vi "Server.vi"() -> ()   [LabVIEW 2013, in "OPC UA Demo.lvlib"]
doc: "Demonstrates the use of the <B>OPC UA Server</B> VIs to programmatically create an OPC UA server."
uses:
  OPC UA Demo.lvlib
  <vilib>/OPCUA/server/subVI/supported security policies.ctl
  <vilib>/OPCUA/server/Write Int32.vi
  <vilib>/OPCUA/server/Read Int32.vi
  <vilib>/OPCUA/NI OPC UA Server.lvlib
  <vilib>/OPCUA/NI OPC UA Utility.lvlib
panel:
  out "appended array":path[](array[path])
  out "certificate path":path
  in  "supported security policies (None)":T1={"None"=TRUE, "Sign with Basic128Rsa125"=TRUE, "Sign and Encrypt with Basic128Rsa125"=TRUE, "Sign with Basic256"=TRUE, "Sign and Encrypt with Basic256"=TRUE}
  out "Device.Node.Set Point":i32
  out "Device.Node":i32
  out "server endpoint URL":string
  out "error out":errorcluster
  in  "stop":bool
  # "Overview: Demonstrates the use of the OPC UA Server VIs to programmatically create an OPC UA server.\nRequirements: \n1. LabVIEW Datalogging and Supervisory Control Module or LabVIEW Real-Time Module\n2. (Real-Time Module) RT target\nInstructions:\nRun the VI."
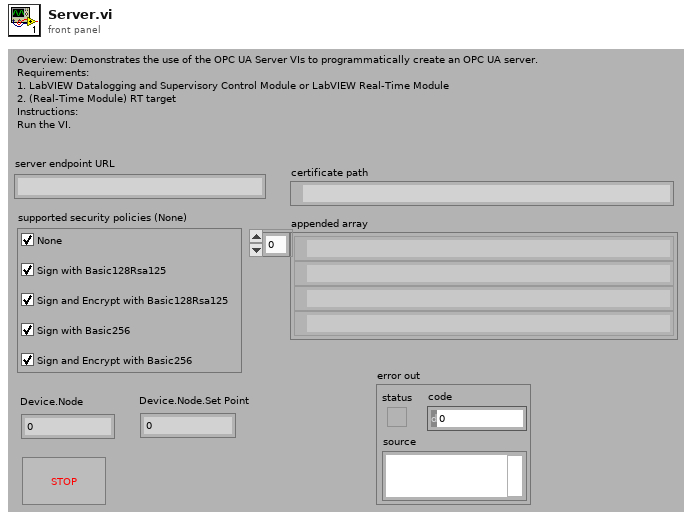
[diagram p1: front panel]
types:
  T1 = typedef "supported security policies.ctl" = cluster{"None":bool, "Sign with Basic128Rsa125":bool, "Sign and Encrypt with Basic128Rsa125":bool, "Sign with Basic256":bool, "Sign and Encrypt with Basic256":bool}
  T2 = cluster{"name":string, "data type":u16, "access level":u16, "description":string}
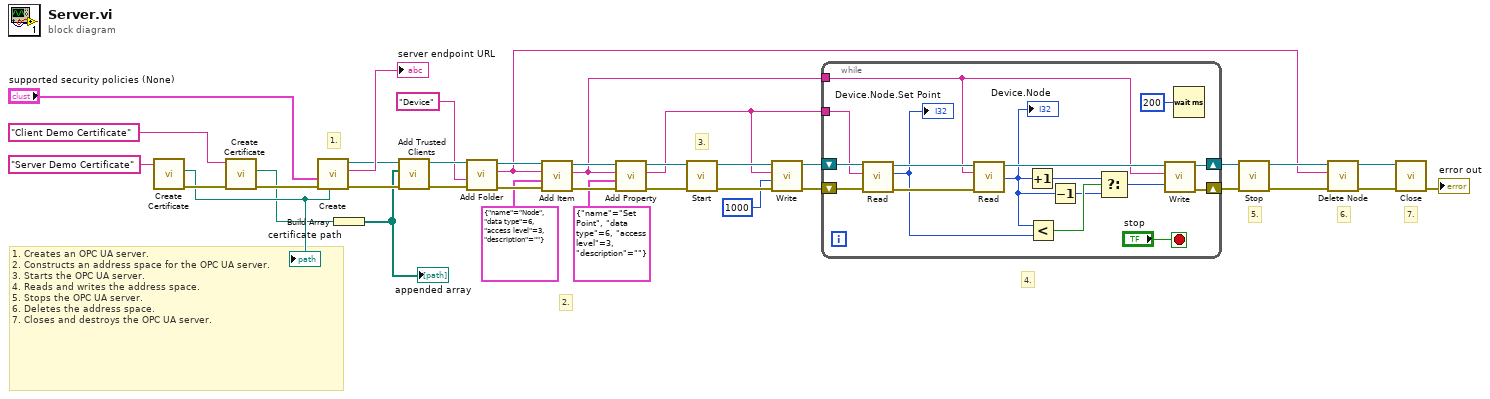
[diagram p0: block diagram]
diagram:
  # "1. Creates an OPC UA server.\n2. Constructs an address space for the OPC UA server.\n3. Starts the OPC UA server.\n4. Reads and writes the address space.\n5. Stops the OPC UA server.\n6. Deletes the address space.\n7. Closes and destroys the OPC UA server."
  # "7."
  # "6."
  # "5."
  # "4."
  # "3."
  # "2."
  # "1."
  n1 = call <vilib>:"Create Certificate.vi"("certificate name in"="Server Demo Certificate") -> ("error out"=w8:errorcluster, "certificate path"=w4:path)  [unwired: 7 in, 2 out]
  "certificate path" <- w4
  n2 = call <vilib>:"Create Certificate.vi"("error in (no error)"=w8, "certificate name in"="Client Demo Certificate") -> ("error out"=w6:errorcluster, "certificate path"=w3:path)  [unwired: 6 in, 2 out]
  n3 = call <vilib>:"Create.vi"("server certificate file"=w4, "error in (no error)"=w6, "supported security policies (None)"="supported security policies (None)") -> ("error out"=w11:errorcluster, "server endpoint URL"=→"server endpoint URL":string, "OPC UA server refnum out"=w13:refnum<k21>)  [unwired: 6 in]
  n4 = Build Array(w3) -> (w7:path[])
  "appended array" <- w7
  n5 = call <vilib>:"Add Trusted Clients.vi"("error in (no error)"=w11, "trusted client certificates"=w7, "OPC UA server refnum in"=w13) -> ("error out"=w10:errorcluster, "OPC UA server refnum out"=w12:refnum<k21>)  [unwired: 7 in]
  n6 = call <vilib>:"Add Folder.vi"("error in (no error)"=w10, "folder name"="Device", "OPC UA server refnum in"=w12) -> ("error out"=w36:errorcluster, "folder path"=w17:string, "OPC UA server refnum out"=w37:refnum<k21>)  [unwired: 5 in]
  n7 = call <vilib>:"Add Item.vi"("error in (no error)"=w36, "item"=T2 {"name"="Node", "data type"=6, "access level"=3, "description"=""}, "parent folder path"=w17, "OPC UA server refnum in"=w37) -> ("error out"=w23:errorcluster, "item path"=w1:string, "OPC UA server refnum out"=w35:refnum<k21>)  [unwired: 4 in]
  n8 = call <vilib>:"Add Property.vi"("error in (no error)"=w23, "property"=T2 {"name"="Set Point", "data type"=6, "access level"=3, "description"=""} ("item"), "item path"=w1, "OPC UA server refnum in"=w35) -> ("error out"=w22:errorcluster, "property path"=w15:string, "OPC UA server refnum out"=w24:refnum<k21>)  [unwired: 4 in]
  n9 = call <vilib>:"Start.vi"("error in (no error)"=w22, "OPC UA server refnum in"=w24) -> ("error out"=w19:errorcluster, "OPC UA server refnum out"=w34:refnum<k21>)  [unwired: 8 in]
  n10 = call-poly <vilib>:"Write.vi"("error in (no error)"=w19, "value"=1000, "node path"=w15, "OPC UA server refnum in"=w34) -> ("error out"=w18:errorcluster, "OPC UA server refnum out"=w20:refnum<k21>)  [unwired: 6 in]
  n11 = while {
    tunnel: w1 -> [w44]
    shift-right: [w50] -> w29
    shift-left: w20 -> [w49]
    shift-right: [w48] -> w27
    shift-left: w18 -> [w52]
    tunnel: w15 -> [w47]
    stop <- "stop" stop-if-true
    n12 = call-poly <vilib>:"Read.vi"("error in (no error)"=w52, "node path"=w47, "OPC UA server refnum in"=w49) -> ("error out"=w45:errorcluster, "value"=w43:i32, "OPC UA server refnum out"=w53:refnum<k21>)  [unwired: 4 in, 2 out]
    "Device.Node.Set Point" <- w43
    n13 = call-poly <vilib>:"Read.vi"("error in (no error)"=w45, "node path"=w44, "OPC UA server refnum in"=w53) -> ("value"=w39:i32, "OPC UA server refnum out"=w46:refnum<k21>)  [unwired: 4 in, 3 out]
    "Device.Node" <- w39
    n14 = Increment(x=w39) -> (x+1=w41:i32)
    n15 = Less?(x=w39, y=w43) -> (x < y?=w42:bool)
    n16 = Decrement(x=w39) -> (x-1=w40:i32)
    n17 = Select(t=w41, s=w42, f=w40) -> (s? t:f=w38:i32)
    n18 = call-poly <vilib>:"Write.vi"("value"=w38, "node path"=w44, "OPC UA server refnum in"=w46) -> ("error out"=w48:errorcluster, "OPC UA server refnum out"=w50:refnum<k21>)  [unwired: 7 in]
    n19 = Wait (ms)(milliseconds to wait=u32 200) -> ()  [unwired: 1 out]
  }
  n20 = call <vilib>:"Stop.vi"("error in (no error)"=w27, "OPC UA server refnum in"=w29) -> ("error out"=w26:errorcluster, "OPC UA server refnum out"=w28:refnum<k21>)  [unwired: 8 in]
  n21 = call <vilib>:"Delete Node.vi"("error in (no error)"=w26, "node path"=w17, "OPC UA server refnum in"=w28) -> ("error out"=w30:errorcluster, "OPC UA server refnum out"=w31:refnum<k21>)  [unwired: 7 in]
  n22 = call <vilib>:"Close.vi"("error in (no error)"=w30, "OPC UA server refnum in"=w31) -> ("error out"=→"error out":errorcluster)  [unwired: 9 in]
